vi "ProcessBufferUpdates.vi"(11 "MockDigitalInput":T1={"BufferUpdateFIFO"="MockDigitalInputCommand"}) -> ()   [LabVIEW 2016, in "FPGAMockDigitalInput.lvlib"]
uses:
  FPGAMockDigitalInput.lvlib
  DataTypes/MockDigitalInputSettings.ctl
  <vilib>/rvi/Emulation/niFpgaGetClockAttributes.vi
  <vilib>/rvi/Emulation/niFpgaSctlEmulationGetInTimedLoop.vi
  <vilib>/rvi/Emulation/niFpgaEmulationReportErrorSimple.vi
  <vilib>/rvi/DataTransferAndStorage/Container/Common/niFpgaContainerExecOnDevCompGetState.vi
  <vilib>/rvi/Emulation/niFpgaEmulationIsFPGAContextNoSignature.vi
  <vilib>/rvi/errors/niFpgaSetErrorForExecOnDevCompSimple.vi
  <vilib>/rvi/eio/common/nirviEmuReportErrorAndStop.vi
  <vilib>/rvi/DataTransferAndStorage/Container/Common/niFpgaContainerGetUniqueNameForEmu.vi
  <vilib>/rvi/FIFO/Fifo_Resource/nirvififoEmulationSetSize.vi
  <vilib>/rvi/FIFO/Fifo_Resource/nirviFifoEmulationQueueMgr.vi
  <instcachedir>/0/nirviFifoEmulationQueueMgr_E5CAEC123FF24DC58D834DCA3CDAA9B5.lvgen/nirviFifoEmulationQueueMgr_E5CAEC123FF24DC58D834DCA3CDAA9B5_000.vi
  <vilib>/rvi/FIFO/Fifo_Resource/nirvififoEmulationDetermineInputValidOut.vi
  <vilib>/rvi/FIFO/Fifo_Resource/nirvififoEmulationCreateLock.vi
  <vilib>/rvi/Emulation/niFpgaProcessEmulError.vi
  <vilib>/rvi/FIFO/Fifo_Resource/nirvififoEmulationObtainLock.vi
  <vilib>/rvi/FIFO/Fifo_Resource/nirvififoEmulationReleaseLock.vi
  <vilib>/rvi/occurrence/nirviWaitOnOccurrenceBase.vi
  <vilib>/rvi/errors/nirviReportUnexpectedCaseInternalError.vi
  <vilib>/rvi/errors/nirviReportUnexpectedCaseInternalError (U32).vi
  <vilib>/Utility/error.llb/Clear Errors.vi
  <vilib>/rvi/interface/RandomDataEmulation/niFpgaRandomDataHandleErrors.vi
  <vilib>/rvi/eio/common/nirviEmuTemplateMethod_errors.vi
  <vilib>/rvi/Emulation/niFpgaCriticalErrorInLSC.vi
  <vilib>/rvi/DataTransferAndStorage/Container/XNode/niFpgaContainer.xnode
  <vilib>/rvi/FIFO/Fifo_Resource/niFpgaFifoEmulationRefIn.vi
  <vilib>/eio/EIONode/EIONode.xnode
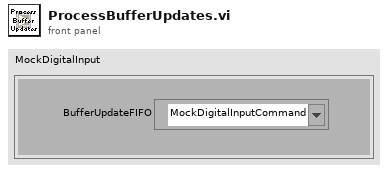
[diagram p1: front panel]
types:
  T1 = typedef "FPGAMockDigitalInput.lvlib/MockDigitalInputSettings.ctl" = cluster{"BufferUpdateFIFO":refnum<k21>}
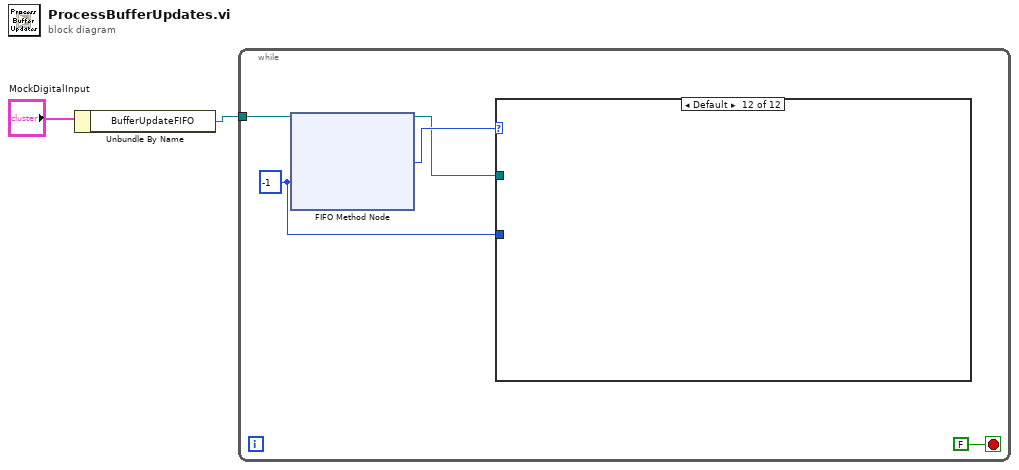
[diagram p0: block diagram]
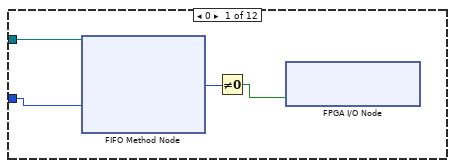
[diagram p2: hidden frame]
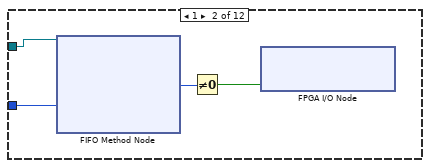
[diagram p3: hidden frame]
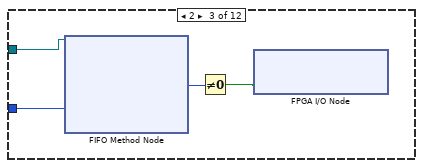
[diagram p4: hidden frame]
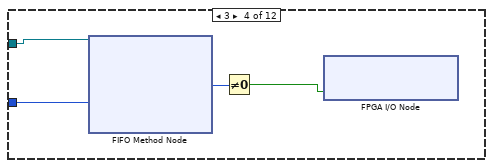
[diagram p5: hidden frame]
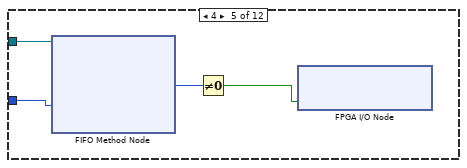
[diagram p6: hidden frame]
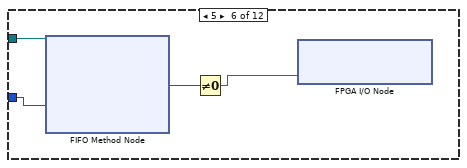
[diagram p7: hidden frame]
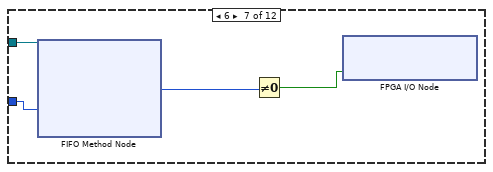
[diagram p8: hidden frame]
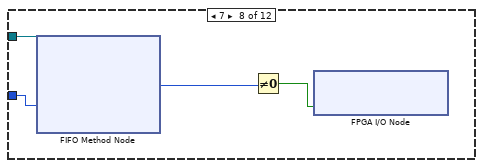
[diagram p9: hidden frame]
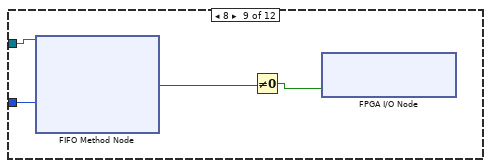
[diagram p10: hidden frame]
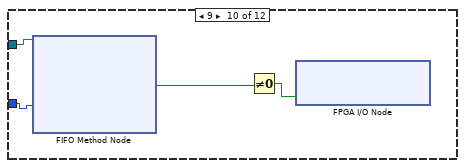
[diagram p11: hidden frame]
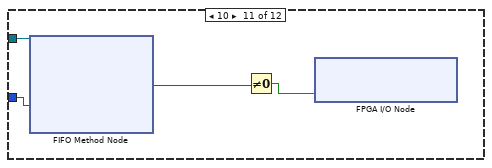
[diagram p12: hidden frame]
diagram:
  n1 = Unbundle By Name("MockDigitalInput") -> ("BufferUpdateFIFO"=w1:refnum<k21>)
  n2 = while {
    tunnel: w1 -> [w6]
    stop <- FALSE stop-if-true
    w3 = -1 ("Timeout")
    n3 = xnode ("FIFO Method Node")("Timeout"=w3, "FIFO In"=w6) -> ("Element"=w5:u8, "FIFO Out"=w4:refnum<k21>)  [unwired: 1 out]
    n4 = case shown="Default" w5 {
      tunnel: w4 -> [w11 w14 w18 w22 w26 w30 w34 w38 w42 w46 w50 _]
      tunnel: w3 -> [w8 w12 w17 w21 w25 w29 w33 w37 w41 w45 w49 _]
      frame 0 {
        n5 = xnode ("FIFO Method Node")("Timeout"=w8, "FIFO In"=w11) -> ("Element"=w10:u8)  [unwired: 2 out]
        n6 = Not Equal To 0?(x=w10) -> (x != 0?=w9:bool)
        n7 = xnode "FPGA I/O Node"("Slot5-DI/DO0"=w9) -> ()  [unwired: 1 in, 1 out]
      }
      frame 1 {
        n8 = xnode ("FIFO Method Node")("Timeout"=w12, "FIFO In"=w14) -> ("Element"=w15:u8)  [unwired: 2 out]
        n9 = Not Equal To 0?(x=w15) -> (x != 0?=w13:bool)
        n10 = xnode "FPGA I/O Node"("Slot5-DI/DO1"=w13) -> ()  [unwired: 1 in, 1 out]
      }
      frame 2 {
        n11 = xnode ("FIFO Method Node")("Timeout"=w17, "FIFO In"=w18) -> ("Element"=w19:u8)  [unwired: 2 out]
        n12 = Not Equal To 0?(x=w19) -> (x != 0?=w16:bool)
        n13 = xnode "FPGA I/O Node"("Slot5-DI/DO2"=w16) -> ()  [unwired: 1 in, 1 out]
      }
      frame 3 {
        n14 = xnode ("FIFO Method Node")("Timeout"=w21, "FIFO In"=w22) -> ("Element"=w23:u8)  [unwired: 2 out]
        n15 = Not Equal To 0?(x=w23) -> (x != 0?=w20:bool)
        n16 = xnode "FPGA I/O Node"("Slot5-DI/DO3"=w20) -> ()  [unwired: 1 in, 1 out]
      }
      frame 4 {
        n17 = xnode ("FIFO Method Node")("Timeout"=w25, "FIFO In"=w26) -> ("Element"=w27:u8)  [unwired: 2 out]
        n18 = Not Equal To 0?(x=w27) -> (x != 0?=w24:bool)
        n19 = xnode "FPGA I/O Node"("Slot5-DI/DO4"=w24) -> ()  [unwired: 1 in, 1 out]
      }
      frame 5 {
        n20 = xnode ("FIFO Method Node")("Timeout"=w29, "FIFO In"=w30) -> ("Element"=w31:u8)  [unwired: 2 out]
        n21 = Not Equal To 0?(x=w31) -> (x != 0?=w28:bool)
        n22 = xnode "FPGA I/O Node"("Slot5-DI/DO5"=w28) -> ()  [unwired: 1 in, 1 out]
      }
      frame 6 {
        n23 = xnode ("FIFO Method Node")("Timeout"=w33, "FIFO In"=w34) -> ("Element"=w35:u8)  [unwired: 2 out]
        n24 = Not Equal To 0?(x=w35) -> (x != 0?=w32:bool)
        n25 = xnode "FPGA I/O Node"("Slot5-DI/DO6"=w32) -> ()  [unwired: 1 in, 1 out]
      }
      frame 7 {
        n26 = xnode ("FIFO Method Node")("Timeout"=w37, "FIFO In"=w38) -> ("Element"=w39:u8)  [unwired: 2 out]
        n27 = Not Equal To 0?(x=w39) -> (x != 0?=w36:bool)
        n28 = xnode "FPGA I/O Node"("Slot5-DI/DO7"=w36) -> ()  [unwired: 1 in, 1 out]
      }
      frame 8 {
        n29 = xnode ("FIFO Method Node")("Timeout"=w41, "FIFO In"=w42) -> ("Element"=w43:u8)  [unwired: 2 out]
        n30 = Not Equal To 0?(x=w43) -> (x != 0?=w40:bool)
        n31 = xnode "FPGA I/O Node"("Slot5-DI/DO8"=w40) -> ()  [unwired: 1 in, 1 out]
      }
      frame 9 {
        n32 = xnode ("FIFO Method Node")("Timeout"=w45, "FIFO In"=w46) -> ("Element"=w47:u8)  [unwired: 2 out]
        n33 = Not Equal To 0?(x=w47) -> (x != 0?=w44:bool)
        n34 = xnode "FPGA I/O Node"("Slot5-DI/DO9"=w44) -> ()  [unwired: 1 in, 1 out]
      }
      frame 10 {
        n35 = xnode ("FIFO Method Node")("Timeout"=w49, "FIFO In"=w50) -> ("Element"=w51:u8)  [unwired: 2 out]
        n36 = Not Equal To 0?(x=w51) -> (x != 0?=w48:bool)
        n37 = xnode "FPGA I/O Node"("Slot5-DI/DO10"=w48) -> ()  [unwired: 1 in, 1 out]
      }
      frame Default {
      }
    }
  }
